vi "Configure Marker.vi"(0 "VISA resource name":refnum<visa-resource-name>, 1 "Enable Marker (T: Enable)":bool=TRUE, 5 "Active Marker (1: Marker 1)":i32(ring)=1 items=["Marker 1"=1, "Marker 2"=2, "Marker 3"=3, "Marker 4"=4, "Marker 5"=5, "Marker 6"=6], 7 "Marker Mode (0: Position)":i32(ring) items=["Position", "Delta", "Off"], 9 "Marker X-Axis Readout (0: Frequency)":i32(ring) items=["Frequency", "Time", "Period"], 11 "error in (no error)":errorcluster, 12 "Marker Position (5E+6 Hz)":dbl=5000000.0) -> (4 "VISA resource name out":refnum<visa-resource-name>, 15 "error out":errorcluster)   [LabVIEW 2022 SP3, in "Agilent N934X Series.lvlib"]
doc: "Configures the marker settings on the spectrum analyzer."
uses:
  <instrlib>/Agilent N934X Series/Agilent N934X Series.lvlib
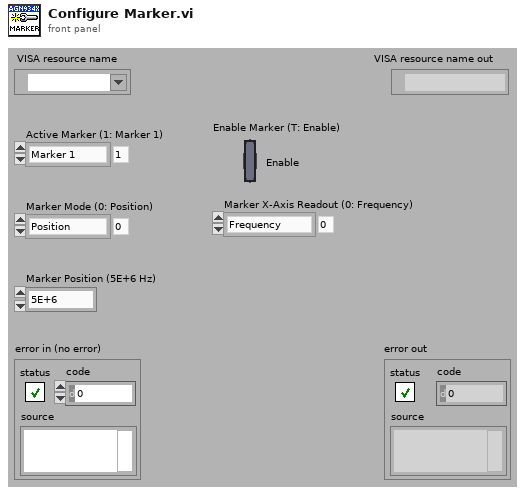
[diagram p1: front panel]
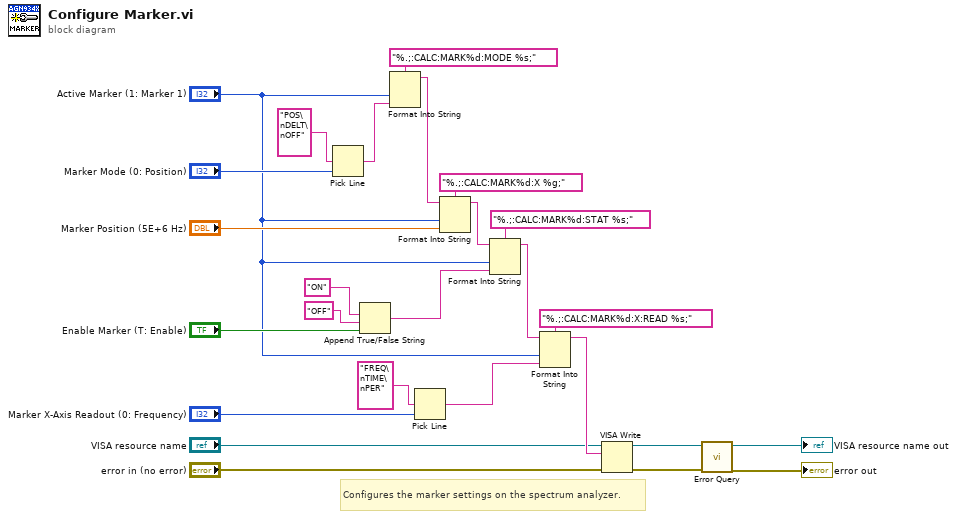
[diagram p0: block diagram]
diagram:
  # "Configures the marker settings on the spectrum analyzer."
  n1 = Pick Line(multi-line string="POS\nDELT\nOFF", line index="Marker Mode (0: Position)") -> (output string=w23:string)  [unwired: 1 in]
  n2 = Append True/False String(1:"Enable Marker (T: Enable)", 2:"OFF", 3:"ON") -> (0:w14:string)  [unwired: 1 in]
  n3 = Format Into String(format string="%.;:CALC:MARK%d:MODE %s;", "Active Marker (1: Marker 1)", w23) -> (resulting string=w22:string)  [unwired: 2 in, 1 out]
  n4 = Pick Line(multi-line string="FREQ\nTIME\nPER", line index="Marker X-Axis Readout (0: Frequency)") -> (output string=w9:string)  [unwired: 1 in]
  n5 = Format Into String(format string="%.;:CALC:MARK%d:X %g;", initial string=w22, "Active Marker (1: Marker 1)", "Marker Position (5E+6 Hz)") -> (resulting string=w16:string)  [unwired: 1 in, 1 out]
  n6 = Format Into String(format string="%.;:CALC:MARK%d:STAT %s;", initial string=w16, "Active Marker (1: Marker 1)", w14) -> (resulting string=w11:string)  [unwired: 1 in, 1 out]
  n7 = Format Into String(format string="%.;:CALC:MARK%d:X:READ %s;", initial string=w11, "Active Marker (1: Marker 1)", w9) -> (resulting string=w8:string)  [unwired: 1 in, 1 out]
  n8 = VISA Write(VISA resource name="VISA resource name", write buffer=w8, error in (no error)="error in (no error)") -> (VISA resource name out=w5:refnum<visa-resource-name>, error out=w4:errorcluster)  [unwired: 1 out]
  n9 = call <instrlib>:"Error Query.vi"("error in (no error)"=w4, "VISA resource name"=w5) -> ("error out"=→"error out":errorcluster, "VISA resource name out"=→"VISA resource name out":refnum<visa-resource-name>)  [unwired: 6 in, 2 out]
